vi "ApplyLayoutToObject.vi"(5 "scaling settings":T1={"scaling factor"={"horizontal"=1.0, "vertical"=1.0}, "scale text"=FALSE} {"scaling factor"."vertical" min=0.0; "scaling factor"."horizontal" min=0.0}, 7 "properties to ignore":variant, 8 "error in (no error)":errorcluster, 10 "GObj Refnum":refnum<vi>, 11 "XControl Layout in":refnum<class "XControl Layout.lvclass">) -> (0 "error out":errorcluster, 3 "XControl Layout out":refnum<class "XControl Layout.lvclass">)   [LabVIEW 2012, in "NI_SE_Front Panel Layout.lvlib" / "XControl Layout.lvclass"]
doc: "Apply layout information to the GObj Refnum."
uses:
  XControl Layout.lvclass
  Scaling Factor_Options.ctl
  XY Scaling Factor.ctl
  Control Layout/Control Layout.lvclass
  XControl Layout.lvclass/XControl Layout.ctl
  Properties To Ignore.vi
  NI_SE_Front Panel Layout.lvlib
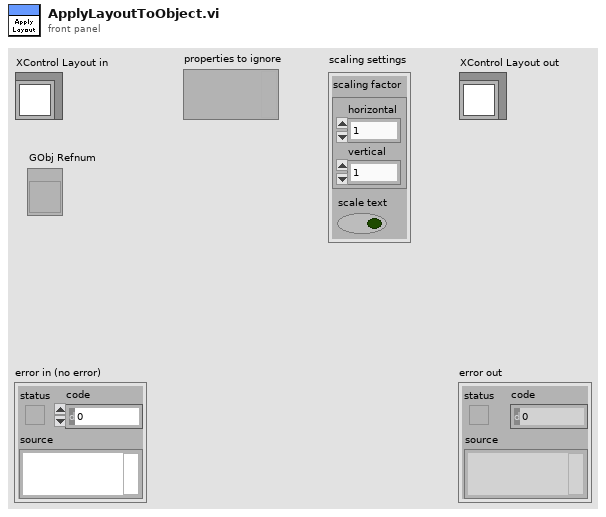
[diagram p1: front panel]
types:
  T1 = typedef "NI_SE_Front Panel Layout.lvlib/Scaling Factor_Options.ctl" = cluster{"scaling factor":T2, "scale text":bool}
  T2 = typedef "NI_SE_Front Panel Layout.lvlib/XY Scaling Factor.ctl" = cluster{"horizontal":dbl, "vertical":dbl}
  T3 = typedef "LVBoundsTypeDef.ctl" = cluster{"Width":u32, "Height":u32}
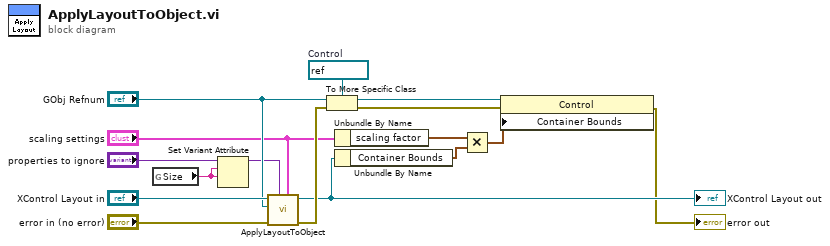
[diagram p0: block diagram]
diagram:
  w7 = refnum<vi> refnum  # Control
  n1 = global read "Properties To Ignore.vi" "Size"() -> (w1:string)
  n2 = Set Variant Attribute(Variant="properties to ignore", name=w1, value=w1) -> (Variant out=w8:variant)  [unwired: 1 in, 2 out]
  n3 = call-parent "ApplyLayoutToObject.vi"("scaling settings"="scaling settings", "properties to ignore"=w8, "error in (no error)"="error in (no error)", "GObj Refnum"="GObj Refnum", "Control Layout in"="XControl Layout in") -> ("error out"=w14:errorcluster, "Control Layout out"=w12:refnum<class "XControl Layout.lvclass">)  [unwired: 5 in]
  "XControl Layout out" <- w12
  n4 = To More Specific Class(target class=w7, reference="GObj Refnum", error in=w14) -> (specific class reference=w6:refnum<vi>, error out=w5:errorcluster)
  n5 = Unbundle By Name("scaling settings") -> ("scaling factor"=w2:T2)
  n6 = Unbundle By Name(w12) -> ("Container Bounds"=w4:T3)
  n7 = Multiply(x=w2, y=w4) -> (x*y=w3:T2)
  n8 = property class="Control"(reference=w6, error in=w5, "Container Bounds"=w3) -> (error out=→"error out":errorcluster)  [unwired: 1 out]
